vi "waitOff.vi"(5 "error in":errorcluster, 8 "queueing interval":i32=100, 10 "Axis #":i8=1 min=1 max=6 step=1, 11 "VISA handle in":refnum<visa-resource-name>) -> (4 "error out 2":errorcluster)   [LabVIEW 2023]
uses:
  truePosition.vi
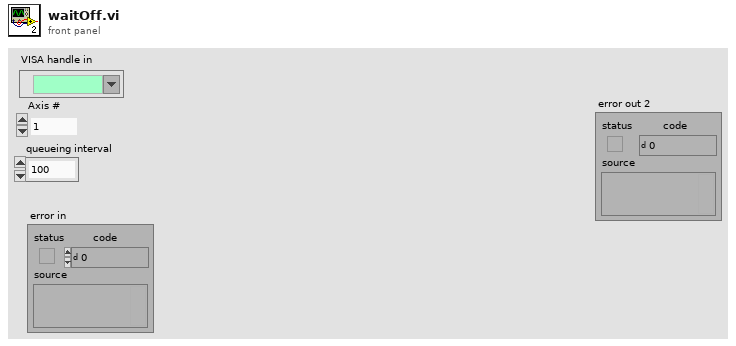
[diagram p1: front panel]
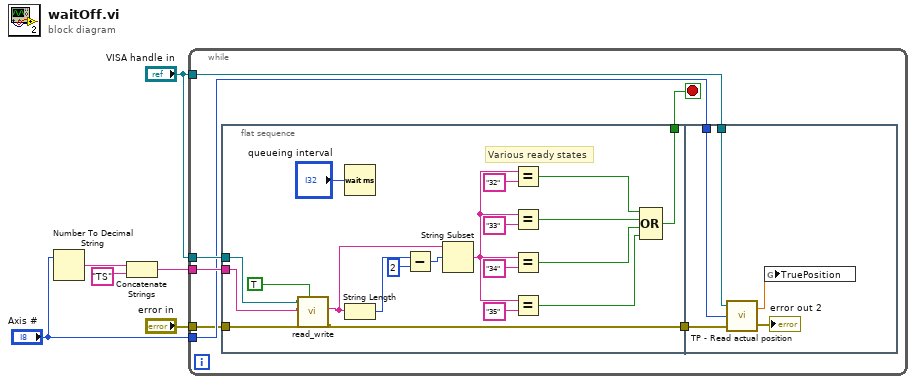
[diagram p0: block diagram]
diagram:
  n1 = Number To Decimal String(number="Axis #") -> (decimal integer string=w6:string)  [unwired: 1 in]
  n2 = Concatenate Strings(w6, "TS" ("Substring")) -> (w4:string)
  n3 = while {
    tunnel: "VISA handle in" -> [w12]
    tunnel: w4 -> [w13]
    tunnel: "error in" -> [w9]
    tunnel: "Axis #" -> [w11]
    tunnel: "VISA handle in" -> [w10]
    stop <- w7 stop-if-true
    n4 = flat-sequence {
      tunnel: w12 -> [w15]
      tunnel: w13 -> [w17]
      tunnel: w9 -> [w19]
      tunnel: [w18] -> w8
      tunnel: [w20] -> w7
      tunnel: w11 -> [w37]
      tunnel: w10 -> [w36]
      tunnel: w8 -> [w34]
      frame #0 {
        # "Various ready states"
        n5 = call "read_write.vi"("Query?"=TRUE, "error in"=w19, "Command"=w17, "VISA handle in"=w15) -> ("error out"=w18:errorcluster, "Response"=w16:string)  [unwired: 2 in, 2 out]
        n6 = Wait (ms)(milliseconds to wait="queueing interval") -> ()  [unwired: 1 out]
        n7 = String Length(string=w16) -> (length=w31:i32)
        n8 = Subtract(x=w31, y=2) -> (x-y=w30:i32)
        n9 = String Subset(string=w16, offset (0)=w30) -> (substring=w25:string)  [unwired: 1 in]
        n10 = Equal?(x=w25, y="32") -> (x = y?=w24:bool)
        n11 = Equal?(x=w25, y="33") -> (x = y?=w23:bool)
        n12 = Equal?(x=w25, y="34") -> (x = y?=w22:bool)
        n13 = Equal?(x=w25, y="35") -> (x = y?=w21:bool)
        n14 = Compound Arithmetic op=OR(w24, w23, w22, w21) -> (w20:bool)
      }
      frame #1 {
        n15 = call "TP - Read actual position.vi"("error in"=w34, "Axis"=w37, "VISA handle in"=w36) -> ("error out"=→"error out 2":errorcluster, "Query the current actual\nposition - read"=w35:dbl)
        n16 = global write "truePosition.vi" "TruePosition"(w35) -> ()
      }
    }
  }
